vi "Drive_Singel Wheel Velocity Tunning.vi"(9 "Smart Motion Parameters":T1={"Max Velocity"=2000.0, "Max Acceleration"=1500.0, "Minimum Velocity Output"=0.0, "Allowed Closed Loop Error"=0.0}, 10 "Velocity PID Constants":T2={"P Gain"=0.0, "I Gain"=0.0, "D Gain"=0.0, "F Gain"=0.0, "I Zone"=0.0, "Min Output"=-1.0, "Max Output"=1.0} {"Max Output" min=-1.0 max=1.0 step=0.01; "Min Output" min=-1.0 max=1.0 step=0.01; "I Zone" step=0.01; "F Gain" step=0.01 format="%.9f"; "D Gain" step=0.01 format="%.9f"; "I Gain" step=0.01 format="%.9f"; "P Gain" min=0.0 step=0.01 format="%.9f"}, 11 "Setpoint":dbl(slide) min=-5000.0 max=5000.0 step=10.0 scale=-5000.0..5000.0) -> ()   [LabVIEW 2023]
uses:
  <vilib>/Rock Robotics/WPI/ThirdParty/REV Robotics/REVLib/Typedef/Spark MAX Smart Motion Parameters.ctl
  <vilib>/Rock Robotics/WPI/ThirdParty/REV Robotics/REVLib/Typedef/Spark MAX Control Type.ctl
  f2715470-5e1a-4aa3-a493-6702d3b8c0f1.vi
  RoboRIO Utilities/Global_STOP.vi
panel:
  in  "Down":bool
  in  "Up":bool
  in  "Step Increment":dbl=10.0 min=-5000.0 max=50000.0 step=10.0
  in  "Reset Time":bool
  in  "milliseconds to wait":u32=50
  in  "Preset Value 3":dbl=4000.0 min=-5000.0 max=50000.0 step=10.0
  in  "Preset Value 2":dbl=2500.0 min=-5000.0 max=50000.0 step=10.0
  in  "Preset Value 1":dbl=1000.0 min=-5000.0 max=50000.0 step=10.0
  in  "Preset 3":bool
  in  "Preset 2":bool
  in  "Preset 1":bool
  in  "Stop":bool
  out "cyle time":dbl
  in  "PIDF Slot (0)":i32
  in  "Device Number":u8=4
  # "Click here to set max"
  # "Click here to set min"
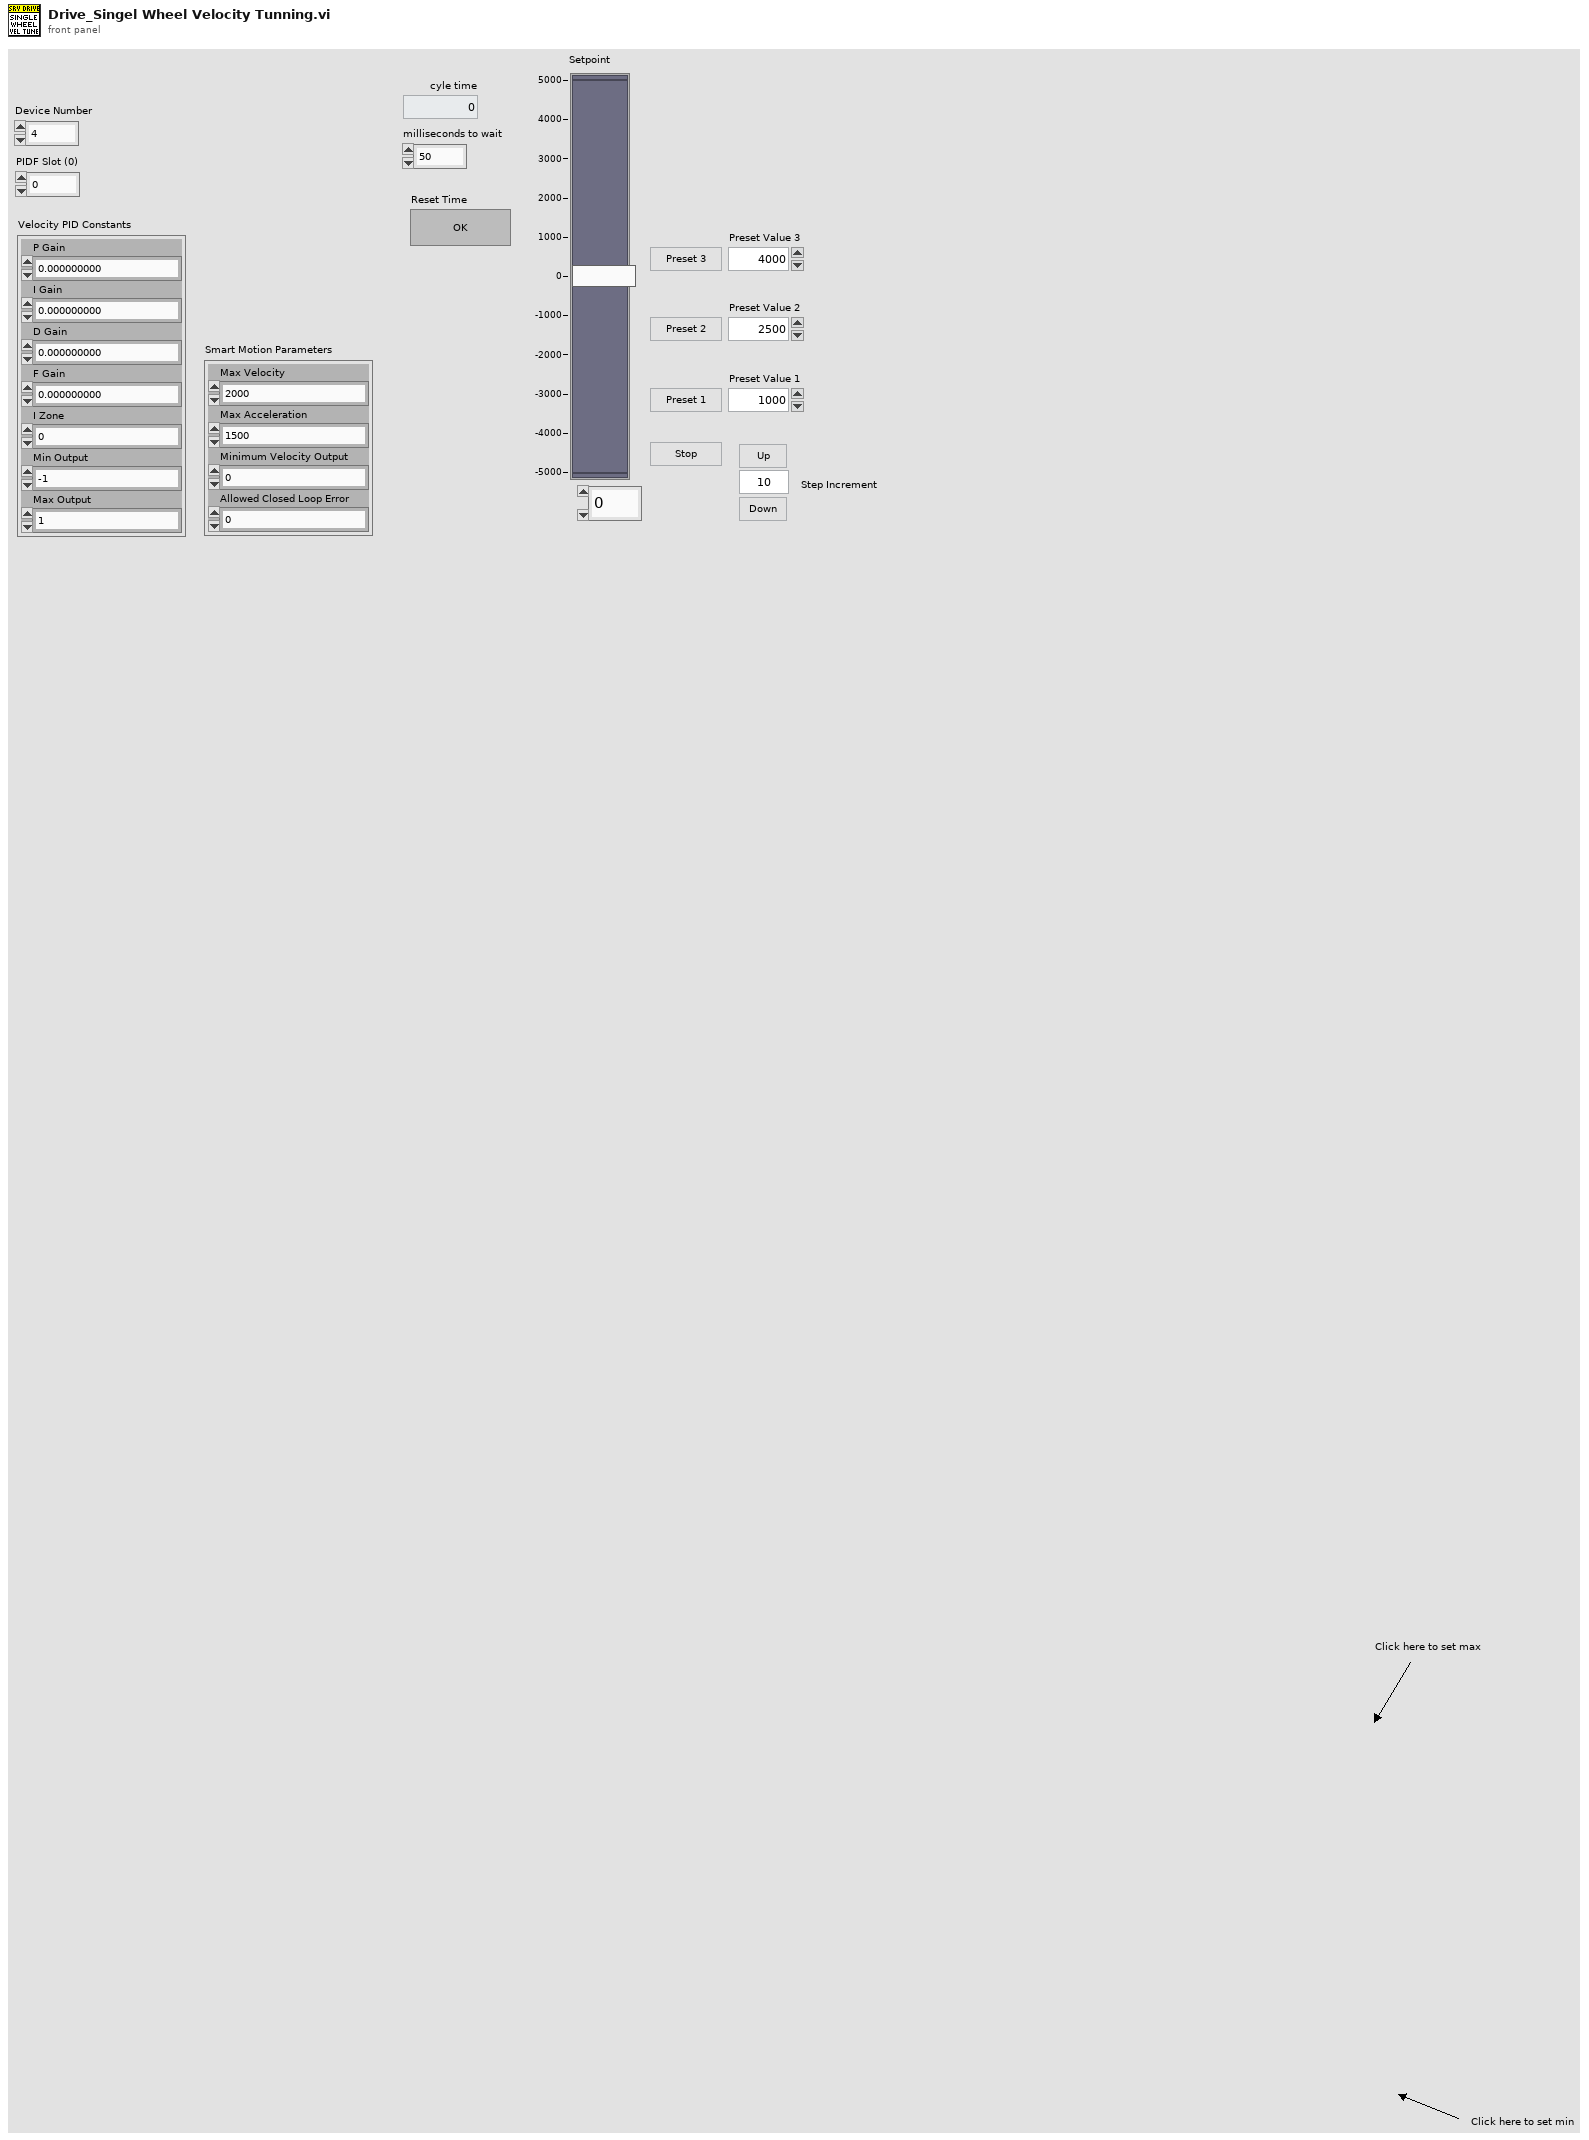
[diagram p1: front panel]
types:
  T1 = typedef "Spark MAX Smart Motion Parameters.ctl" = cluster{"Max Velocity":dbl, "Max Acceleration":dbl, "Minimum Velocity Output":dbl, "Allowed Closed Loop Error":dbl}
  T2 = cluster{"P Gain":dbl, "I Gain":dbl, "D Gain":dbl, "F Gain":dbl, "I Zone":dbl, "Min Output":dbl, "Max Output":dbl}
  T3 = typedef "WPI_MotorControlDeviceRef.ctl" = cluster{"DeviceStatus":errorcluster, "Type":T4, "PWM":cluster{"PWM Channel":T5, "DeadBand":T6}, "CAN":cluster{"Device Number":u8, "SetOutput VI Ref":variant, "GetOutput VI Ref":variant, "Enable VI Ref":variant, "Disable VI Ref":variant, "Data":variant}, "Invert":bool, "DIO PWM":cluster{"PWM \"Enable\" Channel":T5, "DIOChannel":T7, "PWM Rate":dbl}}
  T4 = typedef "WPI_MotorControlType.ctl" = enum16{"PWM", "CAN", "DIO PWM"}
  T5 = typedef "FPGA_DIOPWMChannel.ctl" = enum8{"PWM 0", "PWM 1", "PWM 2", "PWM 3", "PWM 4", "PWM 5", "PWM 6", "PWM 7", "PWM 8", "PWM 9", "PWM MXP 0", "PWM MXP 1", "PWM MXP 2", "PWM MXP 3", "PWM MXP 4", "PWM MXP 5", "PWM MXP 6", "PWM MXP 7", "PWM MXP 8", "PWM MXP 9", "Invalid"}
  T6 = typedef "WPI_PWMDeadband.ctl" = cluster{"Name":string, "maxPositivePwm":i32, "minPositivePwm":i32, "centerPwm":i32, "maxNegativePwm":i32, "minNegativePwm":i32, "angularRange":u16}
  T7 = typedef "FPGA_DIOChannel.ctl" = enum8{"DIO 0", "DIO 1", "DIO 2", "DIO 3", "DIO 4", "DIO 5", "DIO 6", "DIO 7", "DIO 8", "DIO 9", "DIO MXP 0", "DIO MXP 1", "DIO MXP 2", "DIO MXP 3", "DIO MXP 4", "DIO MXP 5", "DIO MXP 6", "DIO MXP 7", "DIO MXP 8", "DIO MXP 9", "DIO MXP 10", "DIO MXP 11", "DIO MXP 12", "DIO MXP 13", "DIO MXP 14", "DIO MXP 15", "SPI Port CS1", "SPI Port CS2", "SPI Port CS3", "SPI Port MISO", "SPI Port MOSI", "Invalid"}
  T8 = typedef "Spark MAX Control Type.ctl" = enum16{"Percent VBus", "Voltage", "Velocity", "Position", "Smart Motion", "Current", "Smart Velocity"}
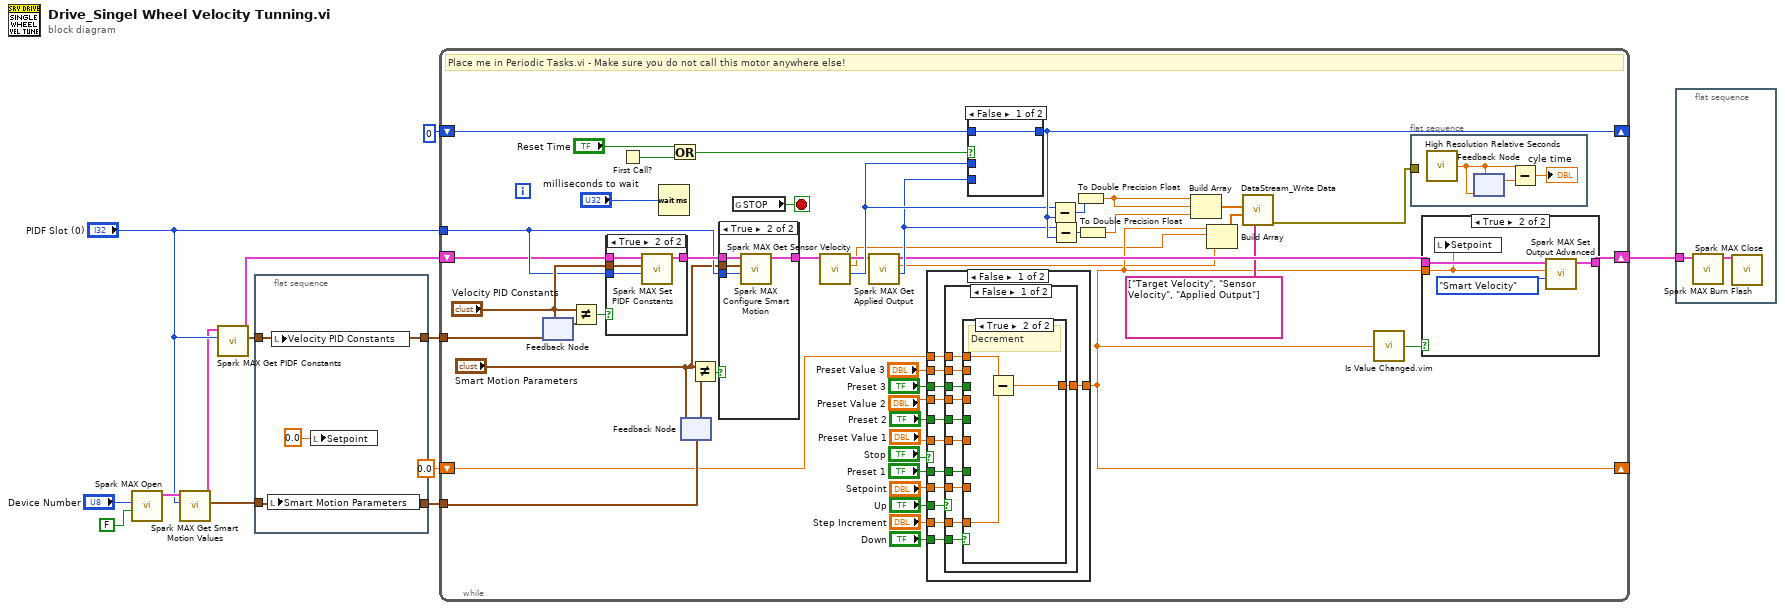
[diagram p0: block diagram]
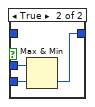
[diagram p2: hidden frame]
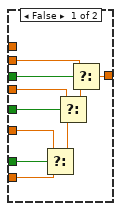
[diagram p4: hidden frame]
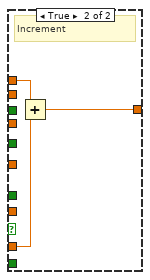
[diagram p5: hidden frame]
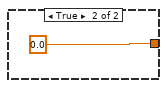
[diagram p6: hidden frame]
diagram:
  n1 = call <vilib>:"Spark MAX Open.vi"("Invert"=FALSE, "Device Number"="Device Number") -> ("MotorControlDeviceRef"=w11:T3)  [unwired: 8 in, 1 out]
  n2 = call <vilib>:"Spark MAX Get Smart Motion Values.vi"("PIDF Slot (0)"="PIDF Slot (0)", "MotorControlDeviceRef"=w11) -> ("Smart Motion Parameters"=w10:T1, "MotorControlDeviceRef"=w5:T3)  [unwired: 7 in, 1 out]
  n3 = call <vilib>:"Spark MAX Get PIDF Constants.vi"("PIDF Slot"="PIDF Slot (0)", "MotorControlDeviceRef"=w5) -> ("PID Constants"=w7:T2, "MotorControlDeviceRef"=w3:T3)  [unwired: 7 in, 1 out]
  n4 = flat-sequence {
    tunnel: w10 -> [w16]
    tunnel: [w16] -> w9
    tunnel: w7 -> [w15]
    tunnel: [w15] -> w6
    frame #0 {
      n5 = local write "Smart Motion Parameters"(w16) -> ()
      n6 = local write "Velocity PID Constants"(w15) -> ()
      n7 = local write "Setpoint"(0.0 ("Setpoint")) -> ()
    }
  }
  n8 = while {
    tunnel: w9 -> [w60]
    tunnel: "PIDF Slot (0)" -> [w54]
    tunnel: w6 -> [w53]
    shift-right: [w51] -> _
    shift-left: u32 0 ("Timestamp") -> [w52]
    shift-right: [w38] -> w2
    shift-left: w3 -> [w37]
    shift-right: [w20] -> _
    shift-left: 0.0 ("Setpoint") -> [w26]
    stop <- w64 stop-if-true
    # "Place me in Periodic Tasks.vi - Make sure you do not call this motor anywhere else!"
    n9 = feedback #1(w53) -> (w55:T2)
    n10 = feedback-in #1("Velocity PID Constants") -> ()
    n11 = Not Equal?(x="Velocity PID Constants", y=w55) -> (x != y?=w57:bool)
    n12 = case shown="True" w57 {
      tunnel: w37 -> [w72 w76]
      tunnel: [w72 w75] -> w62
      tunnel: "Velocity PID Constants" -> [_ w74]
      tunnel: w54 -> [_ w73]
      frame False {
      }
      frame True {
        n13 = call <vilib>:"Spark MAX Set PIDF Constants.vi"("PIDF Slot"=w73, "PID Constants"=w74, "MotorControlDeviceRef"=w76) -> ("MotorControlDeviceRef"=w75:T3)  [unwired: 7 in, 1 out]
      }
    }
    n14 = First Call?() -> (First Call?: T/F=w32:bool)
    n15 = Wait (ms)(milliseconds to wait="milliseconds to wait") -> ()  [unwired: 1 out]
    n16 = Or(x="Reset Time", y=w32) -> (x .or. y?=w34:bool)
    n17 = feedback #2(w60) -> (w58:T1)
    n18 = feedback-in #2("Smart Motion Parameters") -> ()
    n19 = Not Equal?(x="Smart Motion Parameters", y=w58) -> (x != y?=w59:bool)
    n20 = case shown="True" w59 {
      tunnel: w62 -> [w122 w126]
      tunnel: "Smart Motion Parameters" -> [_ w124]
      tunnel: [w122 w125] -> w61
      tunnel: w54 -> [_ w123]
      frame False {
      }
      frame True {
        n21 = call <vilib>:"Spark MAX Configure Smart Motion.vi"("PIDF Slot (0)"=w123, "Smart Motion Parameters"=w124, "MotorControlDeviceRef"=w126) -> ("MotorControlDeviceRef"=w125:T3)  [unwired: 7 in, 1 out]
      }
    }
    n22 = global read "Global_STOP.vi" "STOP"() -> (w64:bool)
    n23 = call <vilib>:"Spark MAX Get Sensor Velocity.vi"("MotorControlDevRef in"=w61) -> ("Timestamp"=w36:u32, "Sensor Velocity"=w19:dbl, "MotorControlDevRef out"=w31:T3)  [unwired: 7 in, 1 out]
    n24 = call <vilib>:"Spark MAX Get Applied Output.vi"("MotorControlDevRef in"=w31) -> ("Timestamp"=w35:u32, "Applied Output"=w18:dbl, "MotorControlDevRef out"=w30:T3)  [unwired: 7 in, 1 out]
    n25 = case shown="False" "Stop" {
      tunnel: "Setpoint" -> [w87 _]
      tunnel: [w84 0.0 ("Setpoint")] -> w20
      tunnel: "Preset 1" -> [w88 _]
      tunnel: "Preset 2" -> [w86 _]
      tunnel: "Preset 3" -> [w85 _]
      tunnel: "Preset Value 3" -> [w83 _]
      tunnel: "Preset Value 2" -> [w82 _]
      tunnel: "Preset Value 1" -> [w81 _]
      tunnel: "Up" -> [w80 _]
      tunnel: "Step Increment" -> [w77 _]
      tunnel: "Down" -> [w79 _]
      tunnel: w26 -> [w78 _]
      frame False {
        n26 = case shown="False" w80 {
          tunnel: w88 -> [w99 _]
          tunnel: w87 -> [w98 _]
          tunnel: w86 -> [w97 _]
          tunnel: w85 -> [w96 _]
          tunnel: [w95 w114] -> w84
          tunnel: w83 -> [w94 _]
          tunnel: w82 -> [w93 _]
          tunnel: w81 -> [w92 _]
          tunnel: w79 -> [w91 _]
          tunnel: w78 -> [w90 w115]
          tunnel: w77 -> [w89 w113]
          frame False {
            n27 = case shown="True" w91 {
              tunnel: w99 -> [w109 _]
              tunnel: w98 -> [w108 _]
              tunnel: w97 -> [w106 _]
              tunnel: w96 -> [w104 _]
              tunnel: [w103 w110] -> w95
              tunnel: w94 -> [w102 _]
              tunnel: w93 -> [w101 _]
              tunnel: w92 -> [w100 _]
              tunnel: w90 -> [_ w112]
              tunnel: w89 -> [_ w111]
              frame False {
                n28 = Select(t=w100, s=w109, f=w108) -> (s? t:f=w107:dbl)
                n29 = Select(t=w101, s=w106, f=w107) -> (s? t:f=w105:dbl)
                n30 = Select(t=w102, s=w104, f=w105) -> (s? t:f=w103:dbl)
              }
              frame True {
                # "Decrement"
                n31 = Subtract(x=w112, y=w111) -> (x-y=w110:dbl)
              }
            }
          }
          frame True {
            # "Increment"
            n32 = Add(x=w115, y=w113) -> (x+y=w114:dbl)
          }
        }
      }
      frame True {
      }
    }
    n33 = case shown="False" w34 {
      tunnel: w36 -> [_ w71]
      tunnel: w35 -> [_ w70]
      tunnel: w52 -> [w68 _]
      tunnel: [w68 w69] -> w51
      frame False {
      }
      frame True {
        n34 = Max & Min(x=w71, y=w70) -> (min(x,y)=w69:u32)  [unwired: 1 out]
      }
    }
    n35 = Subtract(x=w36, y=w51) -> (x-y=w50:u32)
    n36 = Subtract(x=w35, y=w51) -> (x-y=w49:u32)
    n37 = To Double Precision Float(number=w50) -> (double precision float=w23:dbl)
    n38 = To Double Precision Float(number=w49) -> (double precision float=w22:dbl)
    n39 = Build Array(w23, w23, w22) -> (w21:dbl[])
    n40 = Build Array(w20, w19, w18) -> (w17:dbl[])
    n41 = call "DataStream_Write Data.vi"("Header Array"=string[] ["Target Velocity", "Sensor Velocity", "Applied Output"], "Value Array"=w17, "Time Stamp Array"=w21) -> ("Error Out"=w47:errorcluster)  [unwired: 7 in, 1 out]
    n42 = call "Is Value Changed.vim"("value"=w20) -> ("changed or first call?"=w48:bool)
    n43 = flat-sequence {
      tunnel: w47 -> [_]
      frame #0 {
        n44 = call <vilib>:"High Resolution Relative Seconds.vi"() -> ("relative seconds"=w66:dbl)
        n45 = feedback-in #3(w66) -> ()
        n46 = feedback #3(w66) -> (w67:dbl)
        n47 = Subtract(x=w66, y=w67) -> (x-y=→"cyle time":dbl)
      }
    }
    n48 = case shown="True" w48 {
      tunnel: w30 -> [w117 w121]
      tunnel: w20 -> [_ w119]
      tunnel: [w117 w118] -> w38
      frame False {
      }
      frame True {
        n49 = local write "Setpoint"(w119) -> ()
        n50 = call <vilib>:"Spark MAX Set Output Advanced.vi"("Control Mode"=Spark_MAX_Control_Type."Smart Velocity", "Setpoint"=w119, "MotorControlDevRef"=w121) -> ("MotorControlDevRef"=w118:T3)  [unwired: 7 in, 1 out]
      }
    }
  }
  n51 = flat-sequence {
    tunnel: w2 -> [w128]
    frame #0 {
      n52 = call <vilib>:"Spark MAX Burn Flash.vi"("MotorControlDeviceRef"=w128) -> ("MotorControlDeviceRef"=w127:T3)  [unwired: 9 in, 1 out]
      n53 = call <vilib>:"Spark MAX Close.vi"("MotorControlDeviceRef"=w127) -> ()  [unwired: 10 in, 1 out]
    }
  }
